vi "Actor Core.vi"(8 "error in":errorcluster, 11 "Car Wash Controller in":refnum<class "Sim Wash Display Console.lvclass">) -> (0 "error out":errorcluster, 3 "Actor out":refnum<class "Actor.lvclass">)   [LabVIEW 2019, in "Sim Wash Display Console.lvlib" / "Sim Wash Display Console.lvclass"]
doc: "(<B>Filename</B>: Actor Framework.lvlib:Actor.lvclass:Actor Core.vi)\n\nReceives messages to the actor, reacts to them, and initiates any error handling that may shut the actor down.\n\nDescendant classes may override this VI to append parallel tasks for the actor to complete while it handles messages. Overrides use the Call Parent Method node."
uses:
  Sim Wash Display Console.lvclass
  <vilib>/ActorFramework/Stop Msg/Stop Msg.lvclass
  <vilib>/ActorFramework/Actor/Actor.lvclass
  Wash Display Console/Wash Display Console/Wash Display Console.lvclass
  Car Wash Controller/Car Wash Controller Messages/Set Vehicle Position Msg/Set Vehicle Position Msg.lvclass
  C:/Workspace/CLA/Carwasher AF 2nd/Wash Display Console/Wash Display Console/Wash Display Console.lvclass
  C:/Program Files (x86)/National Instruments/LabVIEW 2019/vi.lib/ActorFramework/Actor/Actor.lvclass
  Car Wash Controller/Car Wash Controller Messages/Set Last Step Msg/Set Last Step Msg.lvclass
  Car Wash Controller/Car Wash Controller/Wash Steps.ctl
  Car Wash Controller/Car Wash Controller/Car Wash Controller.lvclass
panel:
  out "Timing Remaining":dbl format="%.2f"
  out "Vehicle Out of Position":bool
  out "Wash Entry":bool
  out "Car Wash Indicators":T1
  # "UI3A\nUI3A1\nUI3A2\nUI3A3"
  # "UI3"
  # "UI3B\nUI3B1\nUI3B2\nUI3B4\nUI3B5"
  # "Mechanical Switch Type"
  # "UI3C\nUI3C1\nUI3C2"
  # "UI3D\nUI3D1"
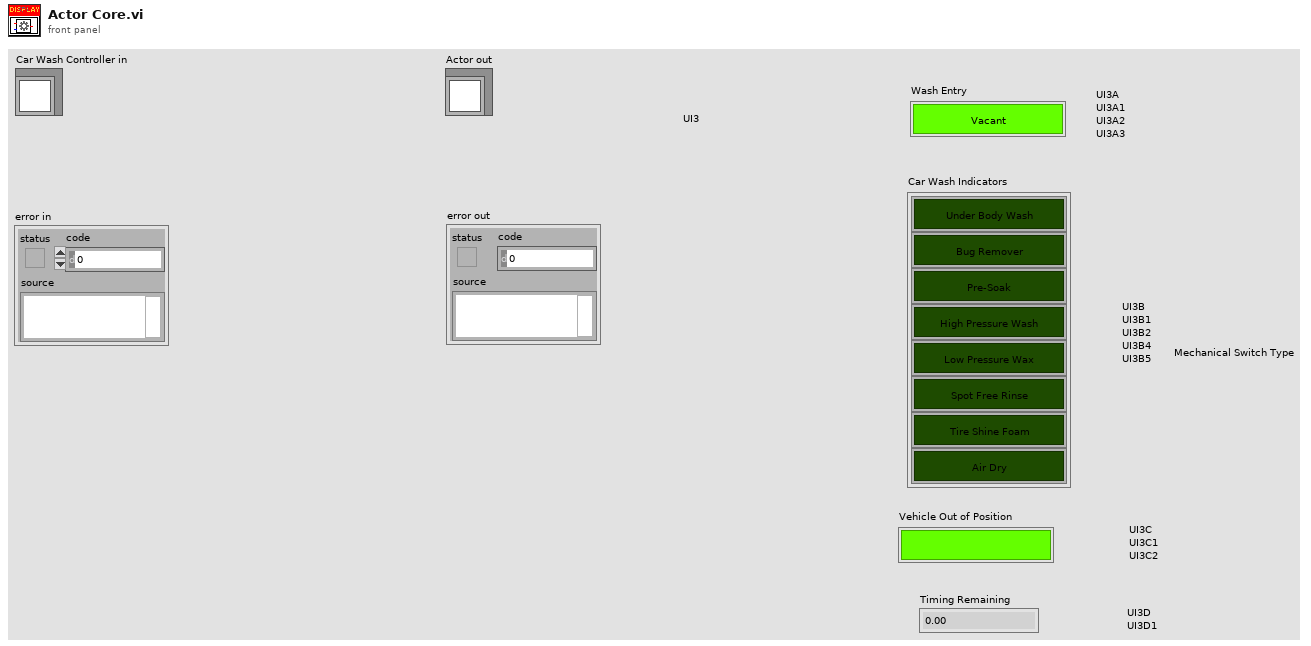
[diagram p1: front panel]
types:
  T1 = typedef "Car Wash Controller.lvlib/Car Wash Controller.lvclass/Wash Steps.ctl" = cluster{"Under Body Wash":bool, "Bug Remover":bool, "Pre-Soak":bool, "High Pressure Wash (Default)":bool, "Low Pressure Wax":bool, "Spot Free Rinse":bool, "Tire Shine Foam":bool, "Air Dry":bool}
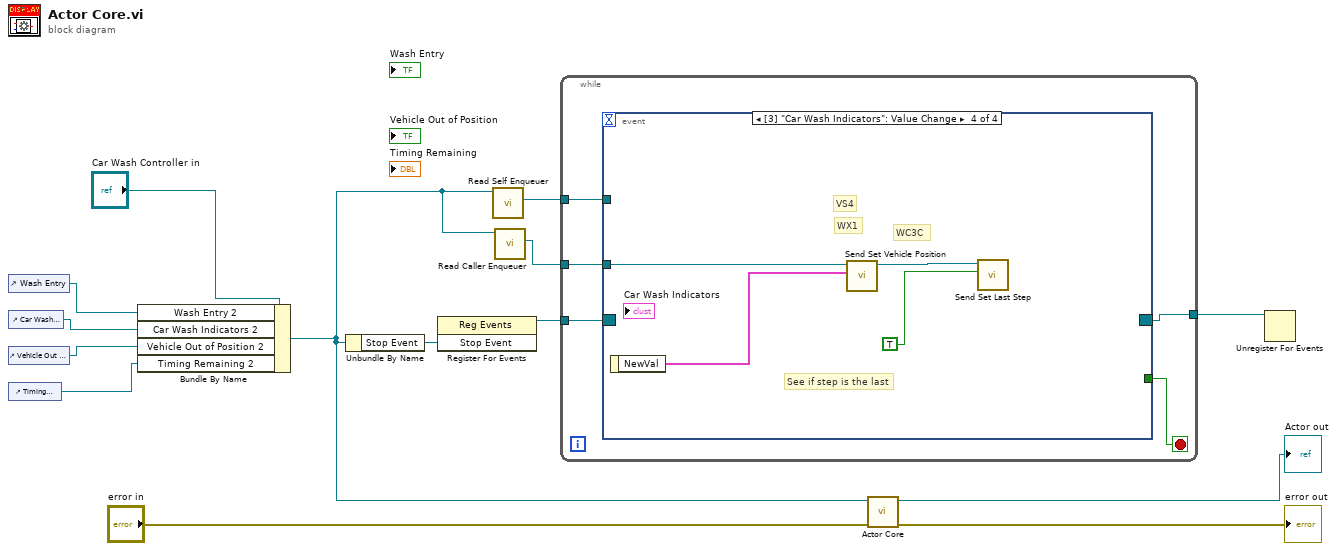
[diagram p0: block diagram]
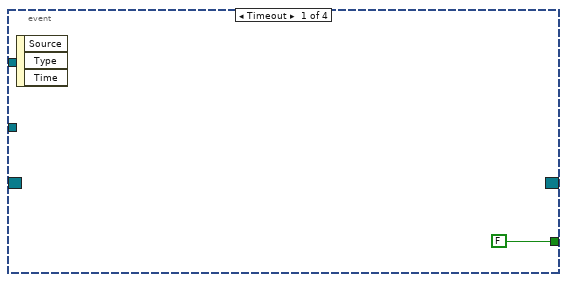
[diagram p2: hidden frame]
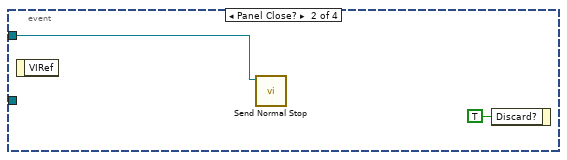
[diagram p3: hidden frame]
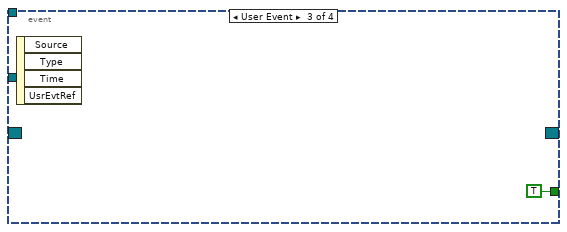
[diagram p4: hidden frame]
diagram:
  n1 = control-ref of="Wash Entry"() -> (w6:refnum<vi>)
  n2 = control-ref of="Car Wash Indicators"() -> (w5:refnum<vi>)
  n3 = control-ref of="Vehicle Out of Position"() -> (w4:refnum<vi>)
  n4 = control-ref of="Timing Remaining"() -> (w3:refnum<vi>)
  n5 = Bundle By Name(cluster="Car Wash Controller in", "Wash Entry 2"=w6, "Car Wash Indicators 2"=w5, "Vehicle Out of Position 2"=w4, "Timing Remaining 2"=w3) -> (w2:refnum<class "Sim Wash Display Console.lvclass">)
  n6 = Unbundle By Name(w2) -> ("Stop Event"=w8:refnum<user-event>)
  n7 = register-events(w8) -> (reference out=w11:refnum<event-registration>)  [unwired: 2 in, 1 out]
  n8 = call <vilib>:"Read Self Enqueuer.vi"("Actor"=w2) -> ("Self Enqueuer"=w9:refnum<class "Message Enqueuer.lvclass">)  [unwired: 10 in]
  n9 = call <vilib>:"Read Caller Enqueuer.vi"("Actor"=w2) -> ("Caller Enqueuer"=w1:refnum<class "Message Enqueuer.lvclass">)  [unwired: 10 in]
  n10 = while {
    tunnel: w11 -> [w18]
    tunnel: [w17] -> w10
    tunnel: w9 -> [w16]
    tunnel: w1 -> [w15]
    stop <- w19 stop-if-true
    n11 = event shown="[3] \"Car Wash Indicators\": Value Change" {
      selector: w18 -> [_ _ _ _]
      dyn-events: [_ _ _ _] -> w17
      timeout: _ -> [_ _ _ _]
      tunnel: [FALSE _ TRUE _] -> w19
      tunnel: w16 -> [_ w21 _ _]
      tunnel: w15 -> [_ _ _ w27]
      event Timeout {
        n12 = event-data() -> ()  [unwired: 1 in, 3 out]
      }
      event Panel Close? {
        n13 = event-data() -> ()  [unwired: 1 in, 1 out]
        n14 = call <vilib>:"Send Normal Stop.vi"("Message Enqueuer"=w21) -> ()  [unwired: 10 in, 1 out]
        n15 = event-data("Discard?"=TRUE) -> ()  [unwired: 1 in, 1 out]
      }
      event User Event {
        n16 = event-data() -> ()  [unwired: 1 in, 4 out]
      }
      event Value Change {
        # "See if step is the last"
        # "WC3C"
        # "WX1"
        # "VS4"
        n17 = event-data() -> ("NewVal"=w26:T1)  [unwired: 1 in]
        n18 = call "Send Set Vehicle Position.vi"("Wash Steps"=w26, "Message Enqueuer"=w27) -> ("Message Enqueuer out"=w24:refnum<class "Message Enqueuer.lvclass">)  [unwired: 8 in, 1 out]
        n19 = call "Send Set Last Step.vi"("Last Step"=TRUE, "Message Enqueuer"=w24) -> ()  [unwired: 8 in, 2 out]
      }
    }
  }
  n20 = call-parent "Actor Core.vi"("error in"="error in", "Actor in"=w2) -> ("error out"=→"error out":errorcluster, "Actor out"=→"Actor out":refnum<class "Actor.lvclass">)  [unwired: 8 in]
  n21 = Unregister For Events(event registration refnum=w10) -> ()  [unwired: 1 in, 1 out]
